vi "TDT ET-Get Hot Block.vi"(0 "TCP":T1, 7 "Timeout (ms)":i32=2000, 11 "error in (no error)":errorcluster) -> (4 "Block Number":i32, 8 "Block Name":string, 10 "Tank Name":string, 15 "error out":errorcluster)   [LabVIEW 2015]
uses:
  Utility VIs/Type Defs/TCP Params.ctl
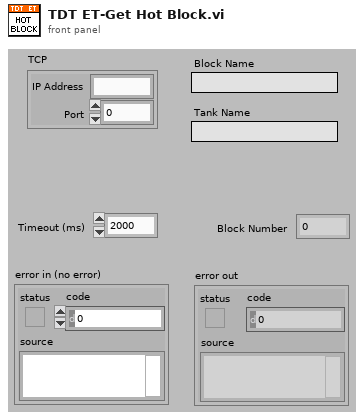
[diagram p1: front panel]
types:
  T1 = typedef "TCP Params.ctl" = cluster{"IP Address":string, "Port":i32}
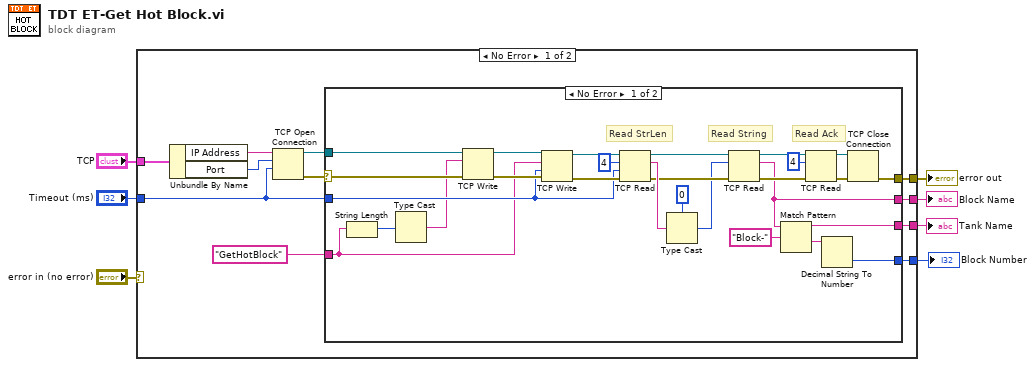
[diagram p0: block diagram]
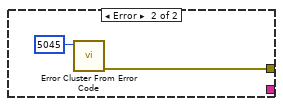
[diagram p2: hidden frame]
diagram:
  n1 = case shown="No Error" "error in (no error)" {
    selector: "error in (no error)" -> [_ w48]
    tunnel: [w12 w48] -> w6
    tunnel: "TCP" -> [w18 _]
    tunnel: "Timeout (ms)" -> [w13 _]
    tunnel: [w10 _] -> w3
    tunnel: [w9 _] -> w2
    tunnel: [w8 _] -> w1
    frame No Error {
      n2 = Unbundle By Name(w18) -> ("IP Address"=w11:string, "Port"=w17:i32)
      n3 = TCP Open Connection(address=w11, remote port or service name=w17, timeout ms (60000)=w13) -> (connection ID=w15:refnum<k5>, error out=w16:errorcluster)  [unwired: 2 in]
      n4 = case shown="No Error" w16 {
        selector: w16 -> [w37 _]
        tunnel: w15 -> [w36 _]
        tunnel: "GetHotBlock" -> [w34 _]
        tunnel: w13 -> [w41 _]
        tunnel: [w40 w47] -> w12
        tunnel: [w22 _] -> w10
        tunnel: [w20 _] -> w9
        tunnel: [w19 _] -> w8
        frame No Error {
          # "Read String"
          # "Read StrLen"
          # "Read Ack"
          n5 = String Length(string=w34) -> (length=w33:i32)
          n6 = Type Cast(x=w33) -> (*(type *) &x=w32:string)  [unwired: 1 in]
          n7 = TCP Write(connection ID=w36, data in=w32, error in (no error)=w37) -> (connection ID out=w35:refnum<k5>, error out=w45:errorcluster)  [unwired: 1 in, 1 out]
          n8 = TCP Write(connection ID=w35, data in=w34, error in (no error)=w45, 9:w41) -> (connection ID out=w43:refnum<k5>, error out=w44:errorcluster)  [unwired: 1 out]
          n9 = TCP Read(connection ID=w43, bytes to read=4, error in (no error)=w44, 9:w41) -> (connection ID out=w30:refnum<k5>, data out=w39:string, error out=w31:errorcluster)  [unwired: 1 in]
          n10 = Type Cast(type=0, x=w39) -> (*(type *) &x=w29:i32)
          n11 = TCP Read(connection ID=w30, bytes to read=w29, error in (no error)=w31) -> (connection ID out=w25:refnum<k5>, data out=w22:string, error out=w27:errorcluster)  [unwired: 2 in]
          n12 = Match Pattern(string=w22, regular expression="Block-") -> (before substring=w19:string, after substring=w21:string)  [unwired: 1 in, 2 out]
          n13 = TCP Read(connection ID=w25, bytes to read=4, error in (no error)=w27) -> (connection ID out=w24:refnum<k5>, error out=w26:errorcluster)  [unwired: 2 in, 1 out]
          n14 = Decimal String To Number(string=w21) -> (number=w20:i32)  [unwired: 2 in, 1 out]
          n15 = TCP Close Connection(connection ID=w24, error in (no error)=w26) -> (error out=w40:errorcluster)  [unwired: 1 in, 1 out]
        }
        frame Error {
          n16 = call <vilib>:"Error Cluster From Error Code.vi"("error code (0)"=5045) -> ("error out"=w47:errorcluster)  [unwired: 8 in]
        }
      }
    }
    frame Error {
    }
  }
  "error out" <- w6
  "Block Name" <- w3
  "Block Number" <- w2
  "Tank Name" <- w1
